vi "Anlyse PSU log.vi"() -> ()   [LabVIEW 2024]
uses:
  <vilib>/Utility/NIReport.llb/Report Type.ctl
  <vilib>/addons/_office/excel.llb/Excel Get Data ([str]).vi
  <vilib>/addons/_office/excel.llb/Excel Get Data ([dbl]).vi
  <vilib>/Utility/NIReport.llb/NI_report.lvclass
  <vilib>/Utility/NIReport.llb/NI_ReportGenerationCore.lvlib
  <vilib>/Utility/NIReport.llb/Excel/NI_Excel.lvclass
  <vilib>/addons/_office/NI_ReportGenerationToolkit.lvlib
panel:
  out "Waveform Chart":dbl[][](graph)
  out "data 2":dbl[][](array[numeric]) format="%.2f"
  out "subarray":string[](array[string])
  out "initialized array":i32[](array[numeric])
  in  "Multicolumn Listbox":i32(listbox)
  out "data":string[][](array[string])
  in  "PSU Log File":path
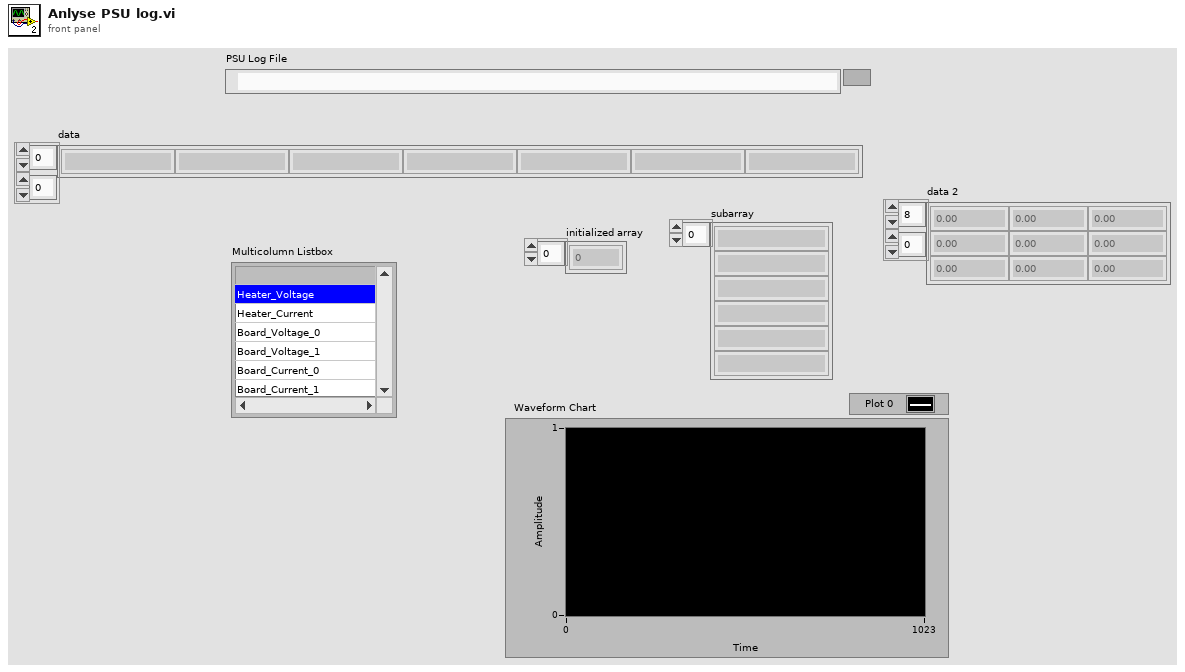
[diagram p1: front panel]
types:
  T1 = typedef "NI_ReportGenerationCore.lvlib/Report Type.ctl" = enum16{"HTML", "Word", "Excel"}
  T2 = cluster{"position (excel)":cluster{"row":i32, "column":i32}, "name (excel)":string, "bookmark (word)":string}
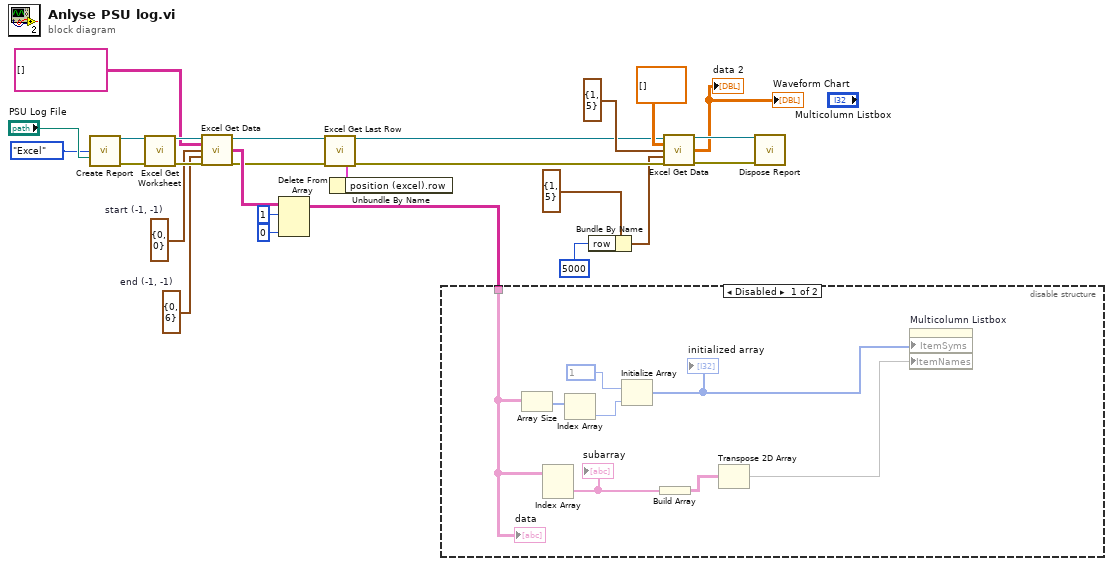
[diagram p0: block diagram]
diagram:
  w18 = cluster{"row":i32, "column":i32} {"row"=0, "column"=6}  # end (-1, -1)
  w19 = cluster{"row":i32, "column":i32} {"row"=0, "column"=0}  # start (-1, -1)
  n1 = call <vilib>:"Create Report.vi"("report type"=Report_Type."Excel", "template (empty)"="PSU Log File") -> ("report out"=w24:refnum<class "NI_report.lvclass">, "error out"=w23:errorcluster)  [unwired: 12 in]
  n2 = call <vilib>:"Excel Get Worksheet.vi"("report in"=w24, "error in (no error)"=w23) -> ("report out"=w22:refnum<class "NI_report.lvclass">, "error out"=w21:errorcluster)  [unwired: 12 in]
  n3 = call-poly <vilib>:"Excel Get Data.vi"("report in"=w22, "data type"=string[][] [], "start (-1, -1)"=w19, "end (-1, -1)"=w18, "error in (no error)"=w21) -> ("report out"=w11:refnum<class "NI_report.lvclass">, "data"=w17:string[][], "error out"=w10:errorcluster)  [unwired: 8 out]
  n4 = Delete From Array(array=w17, length=1, index (col)=0 ("disabled index (col)")) -> (array with subset deleted=w14:string[][])  [unwired: 1 in, 1 out]
  n5 = call <vilib>:"Excel Get Last Row.vi"("report in"=w11, "error in (no error)"=w10) -> ("report out"=w9:refnum<class "NI_report.lvclass">, "MS Office parameters out"=w7:T2, "error out"=w8:errorcluster)  [unwired: 11 in]
  n6 = Unbundle By Name(w7) -> ()  [unwired: 1 out]
  n7 = disable-structure shown="Disabled" {
    disable-tunnel: w14 -> [w32 _]
    frame Disabled {
      n8 = Array Size(array=w32) -> (size(s)=w34:i32[])
      n9 = Index Array(array=w32) -> (element=w29:string[])  [unwired: 2 in]
      "subarray" <- w29
      n10 = Index Array(array=w34) -> (element=w33:i32)  [unwired: 1 in]
      n11 = Initialize Array(1, w33) -> (w30:i32[])
      "initialized array" <- w30
      n12 = Build Array(w29) -> (w28:string[][])
      n13 = Transpose 2D Array(2D array=w28) -> (transposed array=w27:string[][])
      n14 = property on="Multicolumn Listbox" class="MCListbox (strict)"("ItemSyms"=w30, "ItemNames"=w27) -> ()  [unwired: 2 in, 2 out]
      "data" <- w32
    }
    frame Enabled {
    }
  }
  n15 = Bundle By Name(cluster=cluster{"row":i32, "column":i32} {"row"=1, "column"=5} ("end (-1, -1)"), "row"=5000) -> (w5:cluster{"row":i32, "column":i32})
  n16 = call-poly <vilib>:"Excel Get Data.vi"("report in"=w9, "data type"=dbl[][] [], "start (-1, -1)"=cluster{"row":i32, "column":i32} {"row"=1, "column"=5}, "end (-1, -1)"=w5, "error in (no error)"=w8) -> ("report out"=w3:refnum<class "NI_report.lvclass">, "data"=→"data 2" →"Waveform Chart":dbl[][], "error out"=w4:errorcluster)  [unwired: 8 out]
  n17 = call-dynamic "Dispose Report.vi"("report in"=w3, "error in (no error)"=w4) -> ()  [unwired: 13 in, 1 out]
